vi "StringToTilecodes.vi"(6 "SpaceTilecode(206)":u32=206, 11 "String":string) -> (3 "Tilecodes":u32[](array[numeric]))   [LabVIEW 2019, in "RT_Game.lvlib" / "Engine.lvclass"]
uses:
  Engine.lvclass
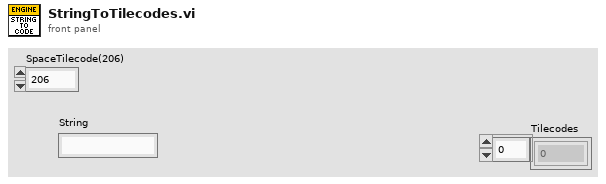
[diagram p1: front panel]
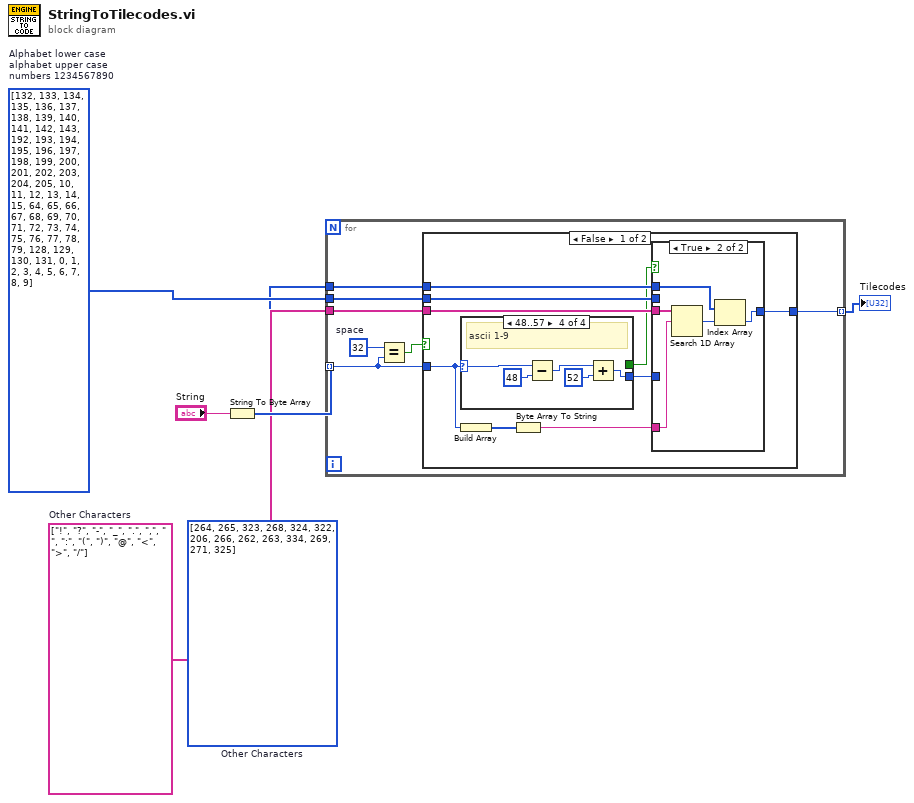
[diagram p0: block diagram]
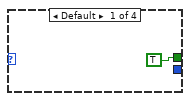
[diagram p2: hidden frame]
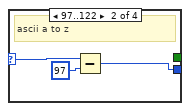
[diagram p3: hidden frame]
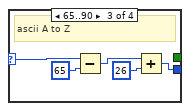
[diagram p4: hidden frame]
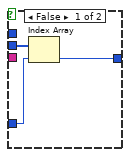
[diagram p5: hidden frame]
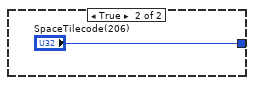
[diagram p6: hidden frame]
diagram:
  w2 = string[] ["!", "?", "-", "_", ".", ",", " ", ":", "(", ")", "@", "<", ">", "/"]  # Other Characters
  w1 = u32[] [264, 265, 323, 268, 324, 322, 206, 266, 262, 263, 334, 269, 271, 325]  # Other Characters
  w4 = u32[] [132, 133, 134, 135, 136, 137, 138, 139, 140, 141, 142, 143, 192, 193, 194, 195, 196, 197, 198, 199, 200, 201, 202, 203, 204, 205, 10, 11, 12, 13, 14, 15, 64, 65, 66, 67, 68, 69, 70, 71, 72, 73, 74, 75, 76, 77, 78, 79, 128, 129, 130, 131, 0, 1, 2, 3, 4, 5, 6, 7, 8, 9]  # Alphabet lower case alphabet upper case numbers 1234567890
  n1 = String To Byte Array(string="String") -> (unsigned byte array=w5:u8[])
  n2 = for {
    tunnel: w5 -> [w8] mode=indexing
    tunnel: w4 -> [w13]
    tunnel: [w12] -> w3 mode=indexing
    tunnel: w2 -> [w10]
    tunnel: w1 -> [w11]
    w7 = u8 32  # space
    n3 = Equal?(x=w7, y=w8) -> (x = y?=w9:bool)
    n4 = case shown="False" w9 {
      tunnel: w13 -> [w22 _]
      tunnel: [w20 "SpaceTilecode(206)"] -> w12
      tunnel: w11 -> [w19 _]
      tunnel: w10 -> [w18 _]
      tunnel: w8 -> [w17 _]
      frame False {
        n5 = case shown="48..57" w17 {
          selector: w17 -> [_ w26 w31 w36]
          tunnel: [_ w24 w27 w32] -> w21
          tunnel: [TRUE _ _ _] -> w14
          frame Default {
          }
          frame 97..122 {
            # "ascii a to z"
            n6 = Subtract(x=w26, y=u8 97) -> (x-y=w24:u8)
          }
          frame 65..90 {
            # "ascii A to Z"
            n7 = Subtract(x=w31, y=u8 65) -> (x-y=w29:u8)
            n8 = Add(x=w29, y=u8 26) -> (x+y=w27:u8)
          }
          frame 48..57 {
            # "ascii 1-9"
            n9 = Subtract(x=w36, y=u8 48) -> (x-y=w34:u8)
            n10 = Add(x=w34, y=u8 52) -> (x+y=w32:u8)
          }
        }
        n11 = Build Array(w17) -> (w16:u8[])
        n12 = Byte Array To String(unsigned byte array=w16) -> (string=w15:string)
        n13 = case shown="True" w14 {
          tunnel: w22 -> [w39 _]
          tunnel: w21 -> [w38 _]
          tunnel: [w37 w40] -> w20
          tunnel: w19 -> [_ w44]
          tunnel: w18 -> [_ w43]
          tunnel: w15 -> [_ w42]
          frame False {
            n14 = Index Array(array=w39, index=w38) -> (element=w37:u32)
          }
          frame True {
            n15 = Search 1D Array(1D array=w43, element=w42) -> (index of element=w41:i32)  [unwired: 1 in]
            n16 = Index Array(array=w44, index=w41) -> (element=w40:u32)
          }
        }
      }
      frame True {
      }
    }
  }
  "Tilecodes" <- w3
